vi "DAQNavi Write (Digital Wfm 1Chan NSamp).vi"(8 "error in (no error)":errorcluster, 9 "timeout":dbl=10.0, 10 "data":digitalwaveform(waveform)={"t0"=timestamp(0 s since 1904-01-01), "dt"=1.0, "Y"={"transitions"=[], "data"=[]}}, 11 "task in":i32) -> (0 "error out":errorcluster, 2 "number of samples written per channel":u32, 3 "task out":i32)   [LabVIEW 2020]
uses:
  <vilib>/Waveform/DWDTOps.llb/DWDT Digital to Binary U8.vi
  DAQNavi_LV.dll
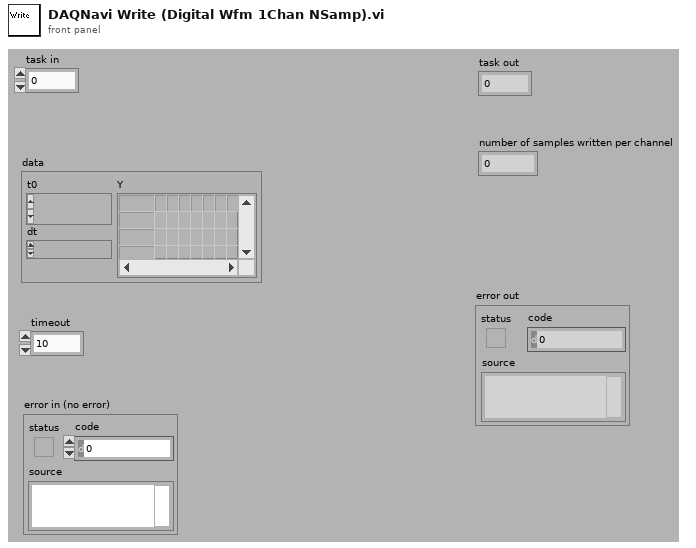
[diagram p1: front panel]
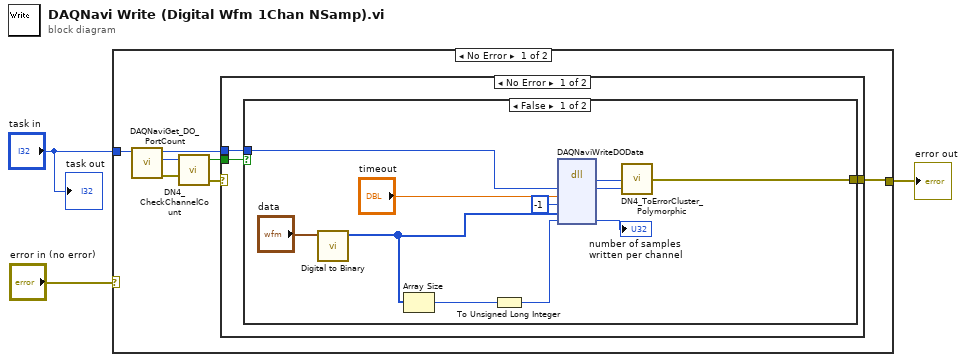
[diagram p0: block diagram]
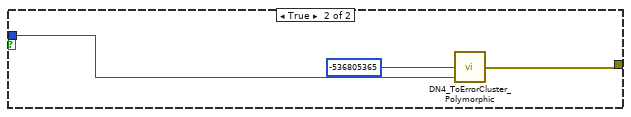
[diagram p2: hidden frame]
diagram:
  n1 = case shown="No Error" "error in (no error)" {
    selector: "error in (no error)" -> [_ w29]
    tunnel: [w9 w29] -> w2
    tunnel: "task in" -> [w10 _]
    frame No Error {
      n2 = call "DAQNaviGet_DO_PortCount.vi"("task in"=w10) -> ("error out"=w7:errorcluster, "port count"=w8:i32, "task out"=w4:i32)  [unwired: 1 in, 7 out]
      n3 = call "DN4_CheckChannelCount.vi"("error out"=w7, "channel count"=w8) -> ("error IO"=w5:errorcluster, "greater than 1?"=w6:bool)  [unwired: 2 out]
      n4 = case shown="No Error" w5 {
        selector: w5 -> [_ w28]
        tunnel: w6 -> [w13 _]
        tunnel: w4 -> [w12 _]
        tunnel: [w11 w28] -> w9
        frame No Error {
          n5 = case shown="False" w13 {
            tunnel: [w20 w26] -> w11
            tunnel: w12 -> [w24 w25]
            frame False {
              n6 = call-poly <vilib>:"Digital to Binary.vi"("digital waveform"="data") -> ("binary array"=w16:u8[])  [unwired: 1 in, 9 out]
              n7 = Array Size(array=w16) -> (size(s)=w19:i32)
              n8 = To Unsigned Long Integer(number=w19) -> (unsigned 32bit integer=w18:u32)
              n9 = dll-call lib="DAQNavi_LV.dll" fn="DAQNaviWriteDOData"("taskID"=w24, "timeout"="timeout", "portBit"=-1, "portData"=w16, "samples"=w18) -> ("return type"=w21:i32, "taskID"=w15:i32, "samples"=→"number of samples written per channel":u32)  [unwired: 6 in, 2 out]
              n10 = call "DN4_ToErrorCluster_Polymorphic.vi"("task id"=w15, "error code"=w21) -> ("error out"=w20:errorcluster)  [unwired: 3 out]
            }
            frame True {
              n11 = call "DN4_ToErrorCluster_Polymorphic.vi"("task id"=w25, "error code"=-536805365 ("error code (0)")) -> ("error out"=w26:errorcluster)  [unwired: 3 out]
            }
          }
        }
        frame Error {
        }
      }
    }
    frame Error {
    }
  }
  "error out" <- w2
  "task out" <- "task in"
